vi "FP_Pane Scrollbars Show Hide.vi"(8 "Error":errorcluster, 9 "Scrollbar Settings":T1, 11 "Pane":refnum<vi>) -> (0 "Error Out":errorcluster, 3 "Pane Out":refnum<vi>)   [LabVIEW 2020]
uses:
  TypeDefs_Utility/Cluster_FP_Scroll Bars Hide Show.ctl
  TypeDefs_Utility/ENUM_FP_Show-Hide Select.ctl
panel:
  in  "Pane Index":i32
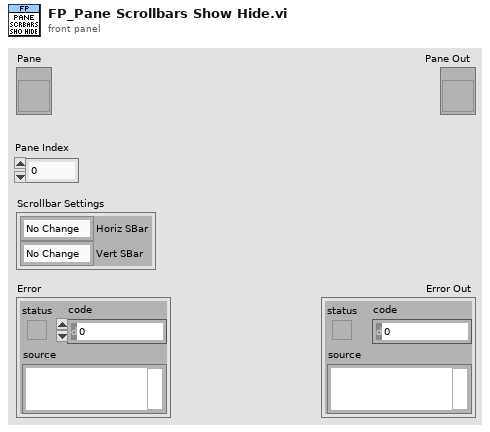
[diagram p1: front panel]
types:
  T1 = typedef "Cluster_FP_Scroll Bars Hide Show.ctl" = cluster{"Horiz SBar":T2, "Vert SBar":T2}
  T2 = typedef "ENUM_FP_Show-Hide Select.ctl" = enum16{"No Change", "Hide", "Show"}
  T3 = enum16{"Always On", "Always Off", "Off While Running"}
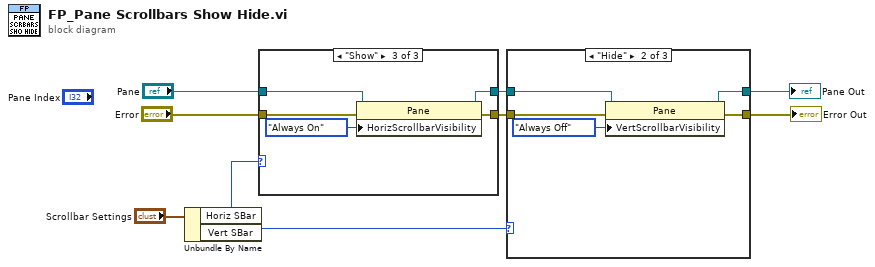
[diagram p0: block diagram]
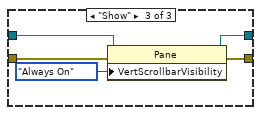
[diagram p3: hidden frame]
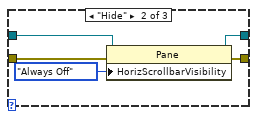
[diagram p5: hidden frame]
diagram:
  n1 = Unbundle By Name("Scrollbar Settings") -> ("Horiz SBar"=w2:T2, "Vert SBar"=w1:T2)
  n2 = case shown="\"Show\"" w2 {
    tunnel: "Pane" -> [w11 w16 w21]
    tunnel: [w11 w15 w20] -> w7
    tunnel: "Error" -> [w10 w14 w19]
    tunnel: [w10 w13 w18] -> w5
    frame "No Change" {
    }
    frame "Hide" {
      n3 = property class="Pane"(reference=w16, error in=w14, "HorizScrollbarVisibility"=T3."Always Off" ("Horizontal Scrollbar Visibility")) -> (reference out=w15:refnum<vi>, error out=w13:errorcluster)
    }
    frame "Show" {
      n4 = property class="Pane"(reference=w21, error in=w19, "HorizScrollbarVisibility"=T3."Always On" ("Horizontal Scrollbar Visibility")) -> (reference out=w20:refnum<vi>, error out=w18:errorcluster)
    }
  }
  n5 = case shown="\"Hide\"" w1 {
    tunnel: [w22 w28 w33] -> w9
    tunnel: w7 -> [w23 w27 w32]
    tunnel: w5 -> [w22 w26 w31]
    tunnel: [w23 w25 w30] -> w3
    frame "No Change" {
    }
    frame "Hide" {
      n6 = property class="Pane"(reference=w27, error in=w26, "VertScrollbarVisibility"=T3."Always Off" ("Vertical Scrollbar Visibility")) -> (reference out=w25:refnum<vi>, error out=w28:errorcluster)
    }
    frame "Show" {
      n7 = property class="Pane"(reference=w32, error in=w31, "VertScrollbarVisibility"=T3."Always On" ("Vertical Scrollbar Visibility")) -> (reference out=w30:refnum<vi>, error out=w33:errorcluster)
    }
  }
  "Error Out" <- w9
  "Pane Out" <- w3
